vi "Send Challenge Response.vi"(8 "error in (no error)":errorcluster, 10 "challenge":string, 11 "Connection in":refnum<class "Connection.lvclass">) -> (0 "error out":errorcluster, 1 "timeout":bool, 2 "Challenge Response":T1, 3 "Connection out":refnum<class "Connection.lvclass">)   [LabVIEW 2013, in "Connection_GOSPL.lvlib" / "Connection.lvclass"]
uses:
  Connection.lvclass
  challenge response -- cluster.ctl
  Connection.lvclass/Connection.ctl
  Store/Store.lvclass
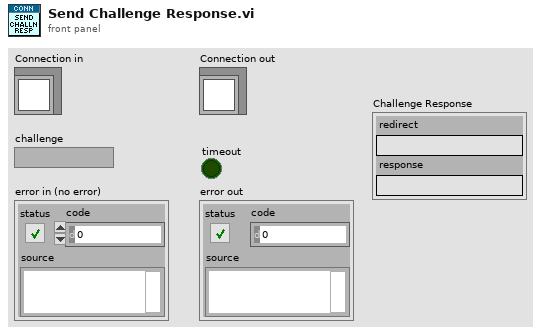
[diagram p1: front panel]
types:
  T1 = typedef "Connection_GOSPL.lvlib/Connection.lvclass/challenge response -- cluster.ctl" = cluster{"redirect":string, "response":string}
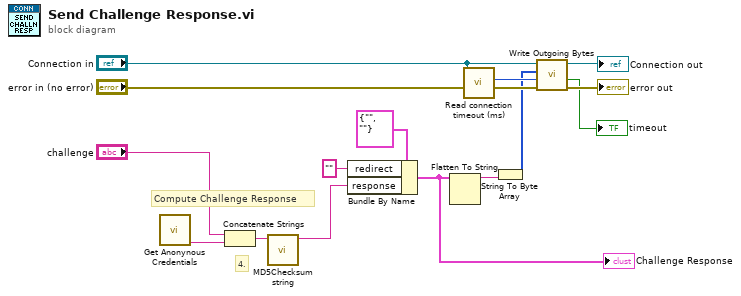
[diagram p0: block diagram]
diagram:
  # "Compute Challenge Response"
  # "4."
  n1 = call "Get Anonynous Credentials.vi"() -> ("Anonymous password"=w8:string)  [unwired: 10 in, 1 out]
  n2 = Concatenate Strings("challenge", w8) -> (w2:string)
  n3 = call <vilib>:"MD5Checksum string.vi"("Message String"=w2) -> ("MD5 message-digest"=w11:string)  [unwired: 10 in]
  n4 = Bundle By Name(cluster=T1 {"redirect"="", "response"=""} ("Challenge Response"), "redirect"="", "response"=w11) -> (w13:T1)
  "Challenge Response" <- w13
  n5 = Flatten To String(anything=w13) -> (data string=w14:string)  [unwired: 3 in, 2 out]
  n6 = call "Read connection timeout (ms).vi"("Connection in"="Connection in") -> ("connection timeout (ms)"=w6:i32)  [unwired: 8 in, 2 out]
  n7 = String To Byte Array(string=w14) -> (unsigned byte array=w4:u8[])
  n8 = call-dynamic "Write Outgoing Bytes.vi"("error in (no error)"="error in (no error)", "timeout (2000 ms)"=w6, "Bytes"=w4, "Connection in"="Connection in") -> ("error out"=→"error out":errorcluster, "timeout"=→"timeout":bool, "Connection out"=→"Connection out":refnum<class "Connection.lvclass">)  [unwired: 5 in]
